vi "Stop Server.vi"(8 "error in":errorcluster, 11 "gRPC Server in":refnum<class "Servicer.lvclass">) -> (0 "error out":errorcluster)   [LabVIEW 2019, in "gRPC-servicer.lvlib" / "Servicer.lvclass"]
uses:
  Servicer.lvclass
  Servicer.lvclass/Servicer.ctl
  gRPC lv Support/grpc-lvsupport/grpc-lvsupport.lvlib
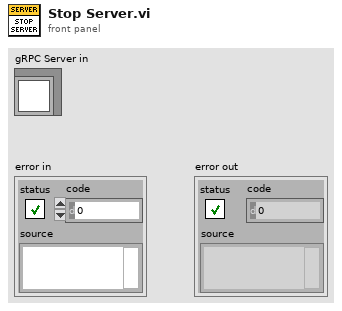
[diagram p1: front panel]
types:
  T1 = typedef "grpc-lvsupport.lvlib/grpcId.ctl" = u64
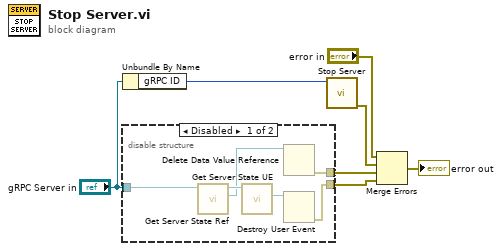
[diagram p0: block diagram]
diagram:
  n1 = Unbundle By Name("gRPC Server in") -> ("gRPC ID"=w1:T1)
  n2 = disable-structure shown="Disabled" {
    disable-tunnel: "gRPC Server in" -> [w11 _]
    disable-tunnel: [w13 _] -> w4
    disable-tunnel: [w12 _] -> w3
    frame Disabled {
      n3 = call "Get Server State Ref.vi"("Template Server in"=w11) -> ("Server State Ref"=w9:refnum<data-value>, "Template Server out"=w10:refnum<class "Servicer.lvclass">)  [unwired: 9 in]
      n4 = call "Get Server State UE.vi"("Template Server in"=w10) -> ("Server Internal State UE"=w8:refnum<user-event>)  [unwired: 9 in, 1 out]
      n5 = Delete Data Value Reference(data value reference=w9) -> (error out=w13:errorcluster)  [unwired: 1 in, 1 out]
      n6 = Destroy User Event(user event=w8) -> (error out=w12:errorcluster)  [unwired: 1 in]
    }
    frame Enabled {
    }
  }
  n7 = call "Stop Server.vi"("gRPCid server in"=w1) -> ("error out"=w5:errorcluster)  [unwired: 10 in]
  n8 = Merge Errors("error in", w5, w4, w3) -> (→"error out":errorcluster)
